vi "ShootTeleOp.vi"(10 "Robot":T1, 11 "Buttons":bool[](array[boolean])) -> ()   [LabVIEW 2015]
uses:
  Robot Type Def.ctl
  Framework/JoystickMappingNamesTypeDef.ctl
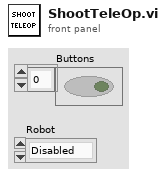
[diagram p1: front panel]
types:
  T1 = typedef "Robot Type Def.ctl" = enum32{"Disabled", "Ghost", "Casper", "Lofty", "Board", "RaceRobot", "Casper 2.0", "Excalibot 2.0"}
  T2 = typedef "JoystickMappingNamesTypeDef.ctl" = enum16{"Shoot Button", "Retrieve Button", "Arm Control", "High Gear", "Low Gear", "Enable PTO", "Disable PTO", "PortC Control", "PortC Up", "PortC Down", "Lift Control", "Drive VBus"}
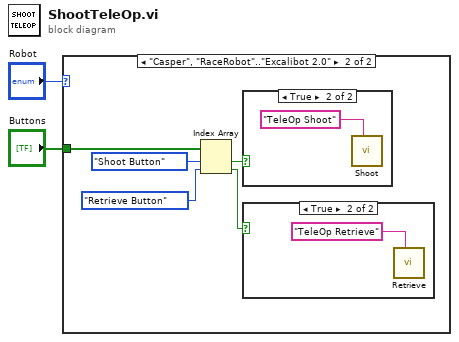
[diagram p0: block diagram]
diagram:
  n1 = case shown="\"Casper\", \"RaceRobot\"..\"Excalibot 2.0\"" "Robot" {
    tunnel: "Buttons" -> [_ w7]
    frame "Disabled", Default {
    }
    frame "Casper", "RaceRobot".."Excalibot 2.0" {
      n2 = Index Array(array=w7, index #1=JoystickMappingNamesTypeDef."Shoot Button" ("Joystick Button Names"), index #2=JoystickMappingNamesTypeDef."Retrieve Button" ("Joystick Button Names")) -> (element #1=w6:bool, element #2=w5:bool)
      n3 = case shown="True" w6 {
        frame False {
        }
        frame True {
          n4 = call "Shoot.vi"("Description"="TeleOp Shoot") -> ()  [unwired: 9 in, 2 out]
        }
      }
      n5 = case shown="True" w5 {
        frame False {
        }
        frame True {
          n6 = call "Retrieve.vi"("Description"="TeleOp Retrieve") -> ()  [unwired: 9 in, 2 out]
        }
      }
    }
  }
